vi "Controller Transform Data.vi"(7 "Mode (Transparent)":enum16{"Transparent", "Replace", "Sum"}(ring), 8 "error in (no error)":errorcluster, 10 "New Data":sgl[](array[numeric]), 11 "Data":dbl[](array[numeric])) -> (0 "error out":errorcluster, 3 "Transformed Data":dbl[](array[numeric]))   [LabVIEW 2011, in "Controller VIs.lvlib"]
uses:
  Controller VIs.lvlib
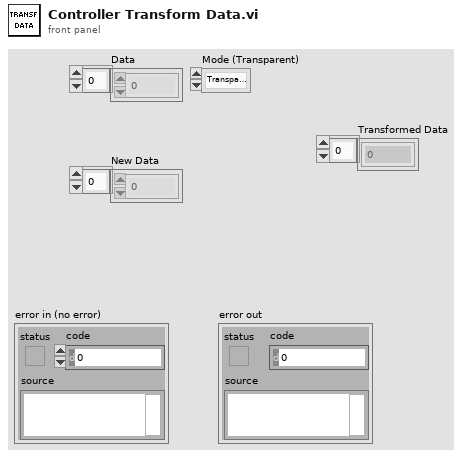
[diagram p1: front panel]
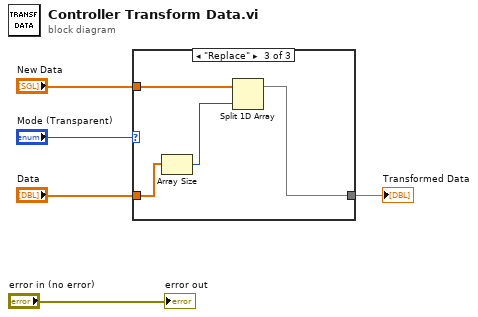
[diagram p0: block diagram]
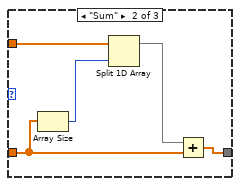
[diagram p3: hidden frame]
diagram:
  n1 = case shown="\"Replace\"" "Mode (Transparent)" {
    tunnel: [w6 w7 w12] -> w4
    tunnel: "Data" -> [w6 w8 w13]
    tunnel: "New Data" -> [_ w11 w15]
    frame "Transparent", Default {
    }
    frame "Sum" {
      n2 = Array Size(array=w8) -> (size(s)=w10:i32)
      n3 = Split 1D Array(array=w11, index=w10) -> (first subarray=w9:sgl[])  [unwired: 1 out]
      n4 = Add(x=w9, y=w8) -> (x+y=w7:dbl[])
    }
    frame "Replace" {
      n5 = Array Size(array=w13) -> (size(s)=w14:i32)
      n6 = Split 1D Array(array=w15, index=w14) -> (first subarray=w12:sgl[])  [unwired: 1 out]
    }
  }
  "Transformed Data" <- w4
  "error out" <- "error in (no error)"
